vi "GetParameters.vi"(0 "Camera Reference in":refnum<k24>, 1 "error in (no error)":errorcluster) -> (2 "2D ExposureMode (Timed Auto HDR Flash)":enum16{"Timed", "Auto", "HDR", "Flash"}(ring), 3 "2D ExposureTime (0.1-999)":dbl=0.1 min=0.1 max=999.0 step=0.1, 4 "2D Gray Value":i32 min=1 max=999 step=1, 5 "2D Auto-Exposure ROI (x, y, width, height)":T2, 6 "2D Tone Mapping":bool, 7 "2D HDR Exposure Count":i32, 8 "2D HDR Exposure Sequence":T1, 9 "3D Exposure Multiplier":i32, 10 "3D Exposure Sequence":T3, 11 "3D Gain (0-16)":dbl, 12 "Depth Range (lower upper)":cluster{"lower":i32, "upper":i32}, 13 "ROI (x, y, width, height)":T2, 14 "Camera Reference out":refnum<k24>, 15 "error out":errorcluster, 16 "PointCloudSurfaceSmoothing (Off Weak Normal Strong)":u8(ring) items=["Off", "Weak", "Normal", "Strong"], 17 "PointCloudNoiseRemoval (Off Weak Normal Strong)":u8(ring) items=["Off", "Weak", "Normal", "Strong"], 18 "PointCloudOutlierRemoval (Off Weak Normal Strong)":u8(ring) items=["Off", "Weak", "Normal", "Strong"], 19 "Stripe Contrast Threshold (0-100)":i32 min=0 max=100 step=1)   [LabVIEW 2023]
uses:
  C:/Program Files/National Instruments/LabVIEW 2025/MechEyeApiNet.dll
  Program Files/National Instruments/LabVIEW 2025/MechEyeApiNet.dll
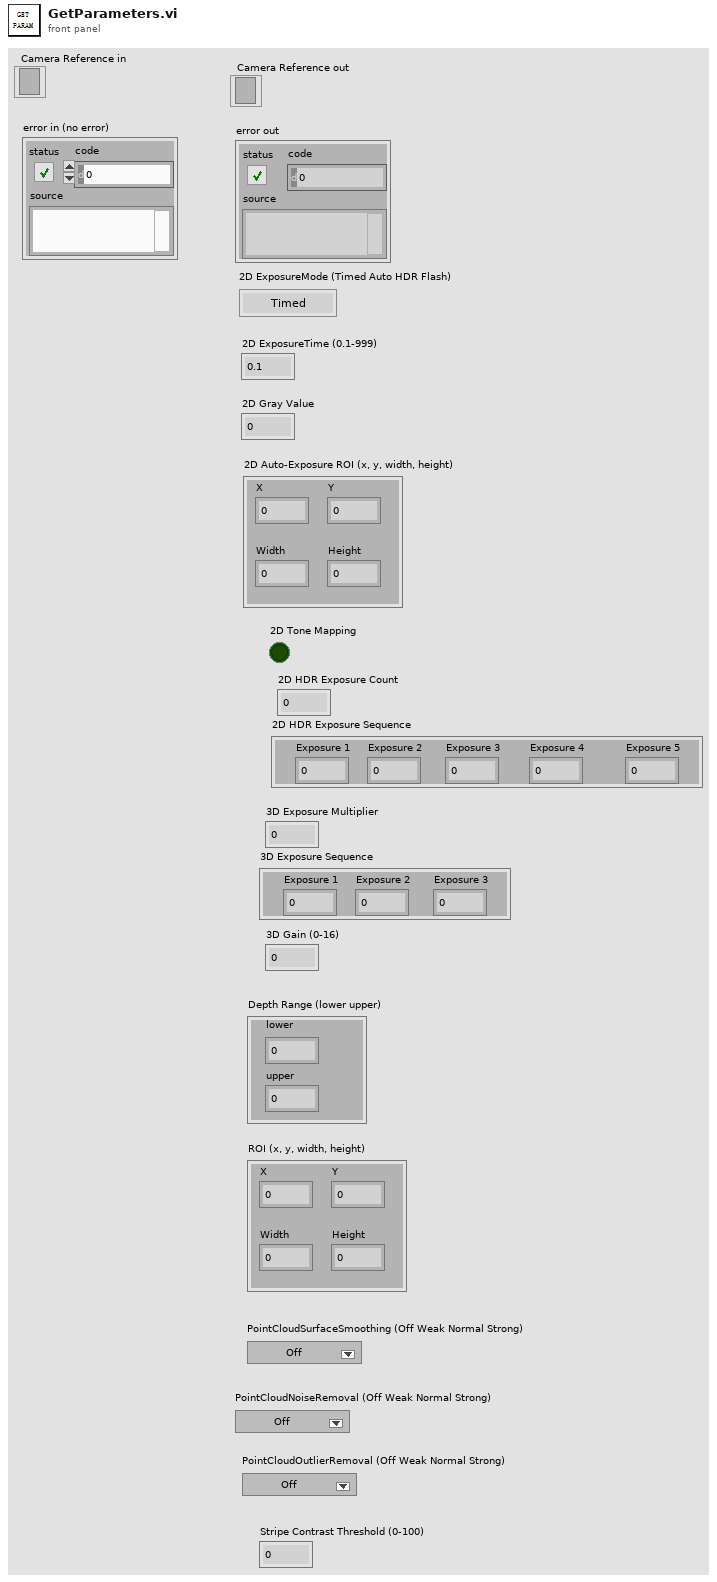
[diagram p1: front panel]
types:
  T1 = cluster{"Exposure 1":dbl, "Exposure 2":dbl, "Exposure 3":dbl, "Exposure 4":dbl, "Exposure 5":dbl}
  T2 = cluster{"X":i32, "Y":i32, "Width":i32, "Height":i32}
  T3 = cluster{"Exposure 1":dbl, "Exposure 2":dbl, "Exposure 3":dbl}
  T4 = cluster{"UpperLeftX":u32, "UpperLeftY":u32, "Width":u64, "Height":u64}
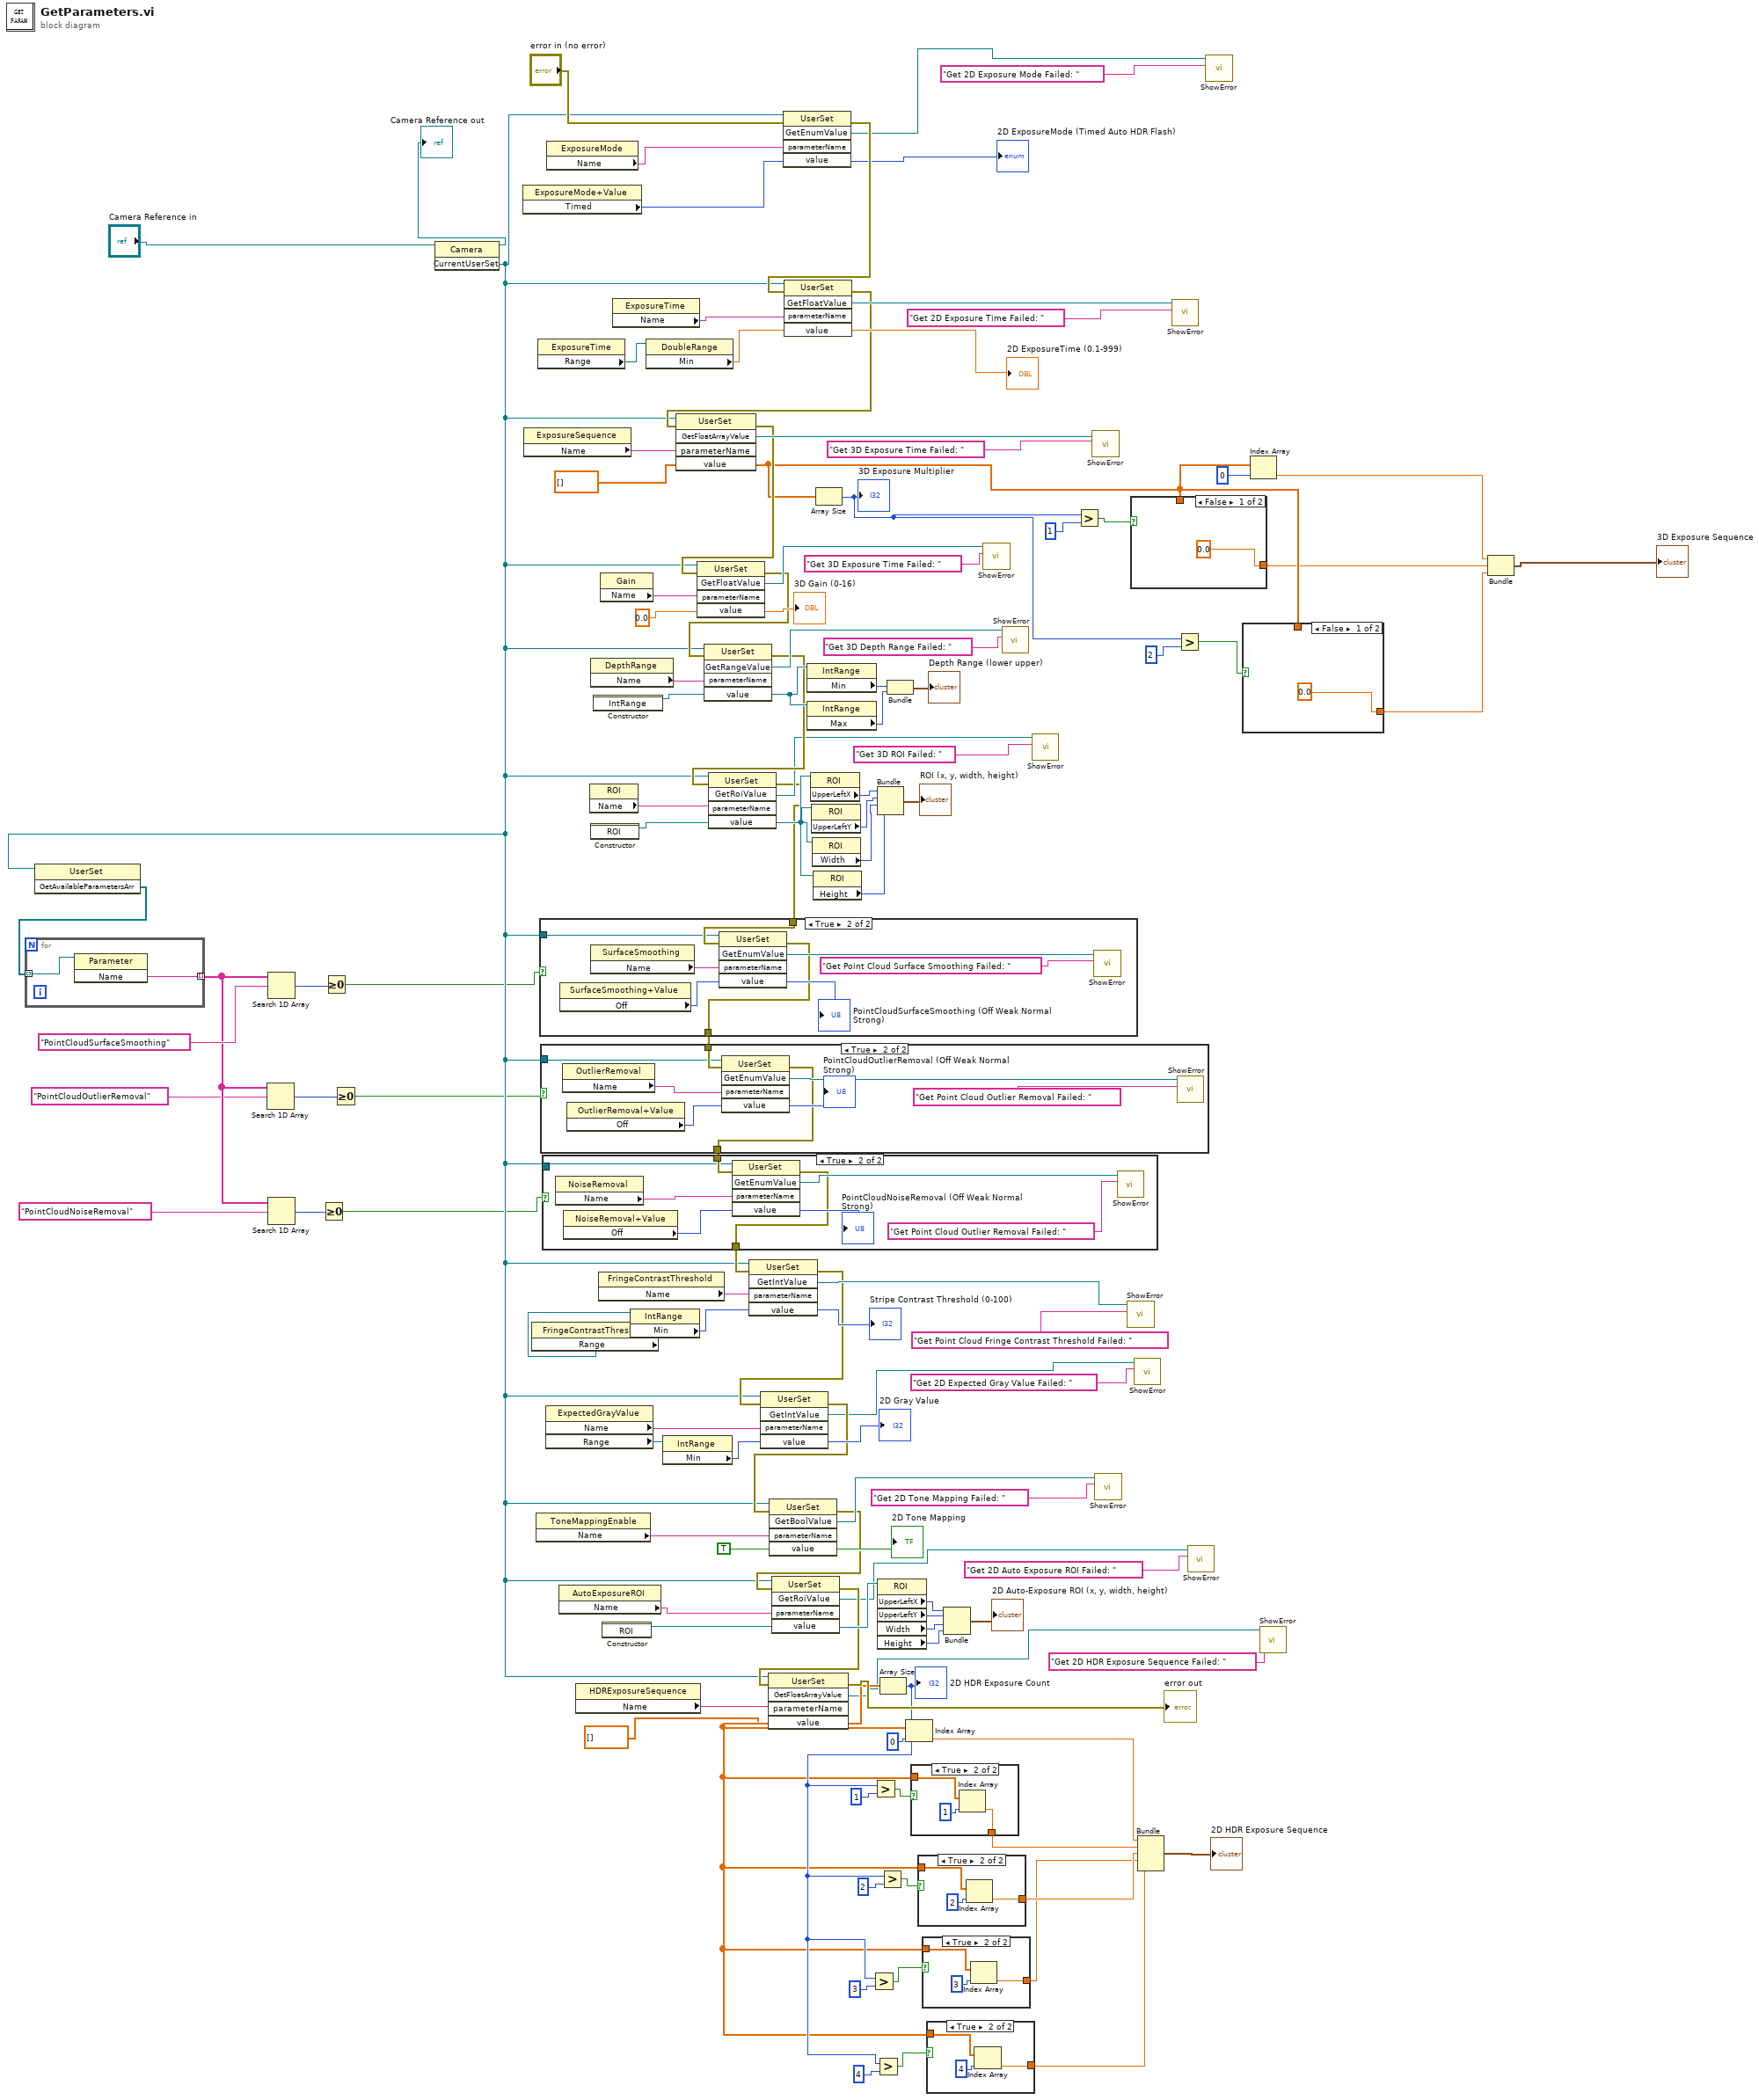
[diagram p0: block diagram]
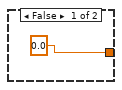
[diagram p5: hidden frame]
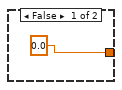
[diagram p6: hidden frame]
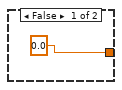
[diagram p7: hidden frame]
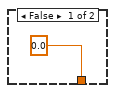
[diagram p8: hidden frame]
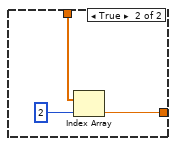
[diagram p9: hidden frame]
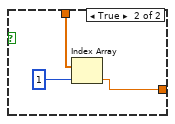
[diagram p10: hidden frame]
diagram:
  n1 = invoke class="Camera" method="CurrentUserSet"(reference="Camera Reference in") -> (reference out=→"Camera Reference out":refnum<k24>, "CurrentUserSet"=w12:refnum<k24>)  [unwired: 2 in, 1 out]
  n2 = invoke class="UserSet" method="GetAvailableParametersArr"(reference=w12) -> ("GetAvailableParametersArr"=w11:refnum<k24>[])  [unwired: 2 in, 2 out]
  n3 = for {
    tunnel: w11 -> [w128] mode=indexing
    tunnel: [w127] -> w7 mode=indexing
    n4 = invoke class="Parameter" method="Name"(reference=w128) -> ("Name"=w127:string)  [unwired: 2 in, 2 out]
  }
  n5 = Search 1D Array(1D array=w7, element="PointCloudOutlierRemoval") -> (index of element=w4:i32)  [unwired: 1 in]
  n6 = Search 1D Array(1D array=w7, element="PointCloudSurfaceSmoothing") -> (index of element=w9:i32)  [unwired: 1 in]
  n7 = Search 1D Array(1D array=w7, element="PointCloudNoiseRemoval") -> (index of element=w3:i32)  [unwired: 1 in]
  n8 = Greater Or Equal To 0?(x=w3) -> (x >= 0?=w1:bool)
  n9 = Greater Or Equal To 0?(x=w9) -> (x >= 0?=w8:bool)
  n10 = Greater Or Equal To 0?(x=w4) -> (x >= 0?=w2:bool)
  n11 = property class="ExposureMode+Value"() -> ("Timed"=w116:i32)  [unwired: 2 in, 2 out]
  n12 = property class="ExposureSequence"() -> ("Name"=w113:string)  [unwired: 2 in, 2 out]
  n13 = property class="FringeContrastThreshold"() -> ("Range"=w74:refnum<k24>)  [unwired: 2 in, 2 out]
  n14 = property class="ToneMappingEnable"() -> ("Name"=w53:string)  [unwired: 2 in, 2 out]
  n15 = property class="ExposureTime"() -> ("Range"=w115:refnum<k24>)  [unwired: 2 in, 2 out]
  n16 = property class="ExpectedGrayValue"() -> ("Name"=w57:string, "Range"=w56:refnum<k24>)  [unwired: 2 in, 2 out]
  n17 = property class="ExposureMode"() -> ("Name"=w120:string)  [unwired: 2 in, 2 out]
  n18 = property class="AutoExposureROI"() -> ("Name"=w45:string)  [unwired: 2 in, 2 out]
  n19 = property class="HDRExposureSequence"() -> ("Name"=w36:string)  [unwired: 2 in, 2 out]
  n20 = property class="ROI"() -> ("Name"=w93:string)  [unwired: 2 in, 2 out]
  n21 = property class="DepthRange"() -> ("Name"=w104:string)  [unwired: 2 in, 2 out]
  n22 = constructor class="ROI"() -> (reference out=w92:refnum<k24>)  [unwired: 3 in, 2 out]
  n23 = constructor class="IntRange"() -> (reference out=w103:refnum<k24>)  [unwired: 3 in, 2 out]
  n24 = property class="FringeContrastThreshold"() -> ("Name"=w75:string)  [unwired: 2 in, 2 out]
  n25 = property class="Gain"() -> ("Name"=w107:string)  [unwired: 2 in, 2 out]
  n26 = constructor class="ROI"() -> (reference out=w38:refnum<k24>)  [unwired: 3 in, 2 out]
  n27 = property class="ExposureTime"() -> ("Name"=w118:string)  [unwired: 2 in, 2 out]
  n28 = property class="IntRange"(reference=w74) -> ("Min"=w73:i32)  [unwired: 1 in, 2 out]
  n29 = property class="DoubleRange"(reference=w115) -> ("Min"=w114:dbl)  [unwired: 1 in, 2 out]
  n30 = property class="IntRange"(reference=w56) -> ("Min"=w55:i32)  [unwired: 1 in, 2 out]
  n31 = invoke class="UserSet" method="GetEnumValue"(reference=w12, error in="error in (no error)", "parameterName"=w120, "value"=w116) -> (error out=w125:errorcluster, "GetEnumValue"=w122:refnum<k24>, "value"=→"2D ExposureMode (Timed Auto HDR Flash)":i32)  [unwired: 1 in, 2 out]
  n32 = invoke class="UserSet" method="GetFloatValue"(reference=w12, error in=w125, "parameterName"=w118, "value"=w114) -> (error out=w96:errorcluster, "GetFloatValue"=w121:refnum<k24>, "value"=→"2D ExposureTime (0.1-999)":dbl)  [unwired: 1 in, 2 out]
  n33 = invoke class="UserSet" method="GetFloatArrayValue"(reference=w12, error in=w96, "parameterName"=w113, "value"=dbl[] [] ("Array")) -> (error out=w95:errorcluster, "GetFloatArrayValue"=w110:refnum<k24>, "value"=w66:dbl[])  [unwired: 1 in, 2 out]
  n34 = invoke class="UserSet" method="GetFloatValue"(reference=w12, error in=w95, "parameterName"=w107, "value"=0.0) -> (error out=w94:errorcluster, "GetFloatValue"=w105:refnum<k24>, "value"=→"3D Gain (0-16)":dbl)  [unwired: 1 in, 2 out]
  n35 = invoke class="UserSet" method="GetRangeValue"(reference=w12, error in=w94, "parameterName"=w104, "value"=w103) -> (error out=w91:errorcluster, "GetRangeValue"=w97:refnum<k24>, "value"=w102:refnum<k24>)  [unwired: 1 in, 2 out]
  n36 = invoke class="UserSet" method="GetRoiValue"(reference=w12, error in=w91, "parameterName"=w93, "value"=w92) -> (error out=w82:errorcluster, "GetRoiValue"=w83:refnum<k24>, "value"=w90:refnum<k24>)  [unwired: 1 in, 2 out]
  n37 = case shown="True" w8 {
    tunnel: w82 -> [w129 w132]
    tunnel: [w129 w131] -> w81
    tunnel: w12 -> [_ w130]
    frame False {
    }
    frame True {
      n38 = property class="SurfaceSmoothing+Value"() -> ("Off"=w135:i32)  [unwired: 2 in, 2 out]
      n39 = property class="SurfaceSmoothing"() -> ("Name"=w136:string)  [unwired: 2 in, 2 out]
      n40 = invoke class="UserSet" method="GetEnumValue"(reference=w130, error in=w132, "parameterName"=w136, "value"=w135) -> (error out=w131:errorcluster, "GetEnumValue"=w133:refnum<k24>, "value"=→"PointCloudSurfaceSmoothing (Off Weak Normal Strong)":i32)  [unwired: 1 in, 2 out]
      n41 = call "ShowError.vi"("String"="Get Point Cloud Surface Smoothing Failed: ", "MMind.Eye.ErrorStatus"=w133) -> ()  [unwired: 10 in]
    }
  }
  n42 = case shown="True" w2 {
    tunnel: w81 -> [w138 w141]
    tunnel: [w138 w140] -> w80
    tunnel: w12 -> [_ w139]
    frame False {
    }
    frame True {
      n43 = property class="OutlierRemoval"() -> ("Name"=w146:string)  [unwired: 2 in, 2 out]
      n44 = property class="OutlierRemoval+Value"() -> ("Off"=w145:i32)  [unwired: 2 in, 2 out]
      n45 = invoke class="UserSet" method="GetEnumValue"(reference=w139, error in=w141, "parameterName"=w146, "value"=w145) -> (error out=w140:errorcluster, "GetEnumValue"=w142:refnum<k24>, "value"=→"PointCloudOutlierRemoval (Off Weak Normal Strong)":i32)  [unwired: 1 in, 2 out]
      n46 = call "ShowError.vi"("String"="Get Point Cloud Outlier Removal Failed: ", "MMind.Eye.ErrorStatus"=w142) -> ()  [unwired: 10 in]
    }
  }
  n47 = case shown="True" w1 {
    tunnel: w80 -> [w147 w150]
    tunnel: [w147 w149] -> w78
    tunnel: w12 -> [_ w148]
    frame False {
    }
    frame True {
      n48 = property class="NoiseRemoval"() -> ("Name"=w155:string)  [unwired: 2 in, 2 out]
      n49 = property class="NoiseRemoval+Value"() -> ("Off"=w154:i32)  [unwired: 2 in, 2 out]
      n50 = invoke class="UserSet" method="GetEnumValue"(reference=w148, error in=w150, "parameterName"=w155, "value"=w154) -> (error out=w149:errorcluster, "GetEnumValue"=w151:refnum<k24>, "value"=→"PointCloudNoiseRemoval (Off Weak Normal Strong)":i32)  [unwired: 1 in, 2 out]
      n51 = call "ShowError.vi"("String"="Get Point Cloud Outlier Removal Failed: ", "MMind.Eye.ErrorStatus"=w151) -> ()  [unwired: 10 in]
    }
  }
  n52 = invoke class="UserSet" method="GetIntValue"(reference=w12, error in=w78, "parameterName"=w75, "value"=w73) -> (error out=w59:errorcluster, "GetIntValue"=w76:refnum<k24>, "value"=→"Stripe Contrast Threshold (0-100)":i32)  [unwired: 1 in, 2 out]
  n53 = invoke class="UserSet" method="GetIntValue"(reference=w12, error in=w59, "parameterName"=w57, "value"=w55) -> (error out=w51:errorcluster, "GetIntValue"=w49:refnum<k24>, "value"=→"2D Gray Value":i32)  [unwired: 1 in, 2 out]
  n54 = invoke class="UserSet" method="GetBoolValue"(reference=w12, error in=w51, "parameterName"=w53, "value"=TRUE) -> (error out=w46:errorcluster, "GetBoolValue"=w47:refnum<k24>, "value"=→"2D Tone Mapping":bool)  [unwired: 1 in, 2 out]
  n55 = invoke class="UserSet" method="GetRoiValue"(reference=w12, error in=w46, "parameterName"=w45, "value"=w38) -> (error out=w37:errorcluster, "GetRoiValue"=w15:refnum<k24>, "value"=w44:refnum<k24>)  [unwired: 1 in, 2 out]
  n56 = invoke class="UserSet" method="GetFloatArrayValue"(reference=w12, error in=w37, "parameterName"=w36, "value"=dbl[] []) -> (error out=→"error out":errorcluster, "GetFloatArrayValue"=w13:refnum<k24>, "value"=w19:dbl[])  [unwired: 1 in, 2 out]
  n57 = property class="IntRange"(reference=w102) -> ("Min"=w101:i32)  [unwired: 1 in, 2 out]
  n58 = property class="IntRange"(reference=w102) -> ("Max"=w100:i32)  [unwired: 1 in, 2 out]
  n59 = property class="ROI"(reference=w90) -> ("UpperLeftX"=w88:u32)  [unwired: 1 in, 2 out]
  n60 = property class="ROI"(reference=w90) -> ("UpperLeftY"=w87:u32)  [unwired: 1 in, 2 out]
  n61 = property class="ROI"(reference=w90) -> ("Width"=w86:u64)  [unwired: 1 in, 2 out]
  n62 = property class="ROI"(reference=w90) -> ("Height"=w85:u64)  [unwired: 1 in, 2 out]
  n63 = Array Size(array=w66) -> (size(s)=w68:i32)
  "3D Exposure Multiplier" <- w68
  n64 = Bundle("UpperLeftX"=w88, "UpperLeftY"=w87, "Width"=w86, "Height"=w85) -> (→"ROI (x, y, width, height)":T4)  [unwired: 1 in]
  n65 = property class="ROI"(reference=w44) -> ("UpperLeftX"=w42:u32, "UpperLeftY"=w41:u32, "Width"=w40:u64, "Height"=w39:u64)  [unwired: 1 in, 2 out]
  n66 = Array Size(array=w19) -> (size(s)=w20:i32)
  "2D HDR Exposure Count" <- w20
  n67 = Greater?(x=w20, y=3) -> (0:w24:bool)
  n68 = Greater?(x=w20, y=1) -> (0:w32:bool)
  n69 = Greater?(x=w20, y=4) -> (0:w21:bool)
  n70 = Greater?(x=w20, y=2) -> (0:w30:bool)
  n71 = Bundle("Min"=w101, "Max"=w100) -> (→"Depth Range (lower upper)":cluster{"Min":i32, "Max":i32})  [unwired: 1 in]
  n72 = Index Array(array=w19, index=0) -> (element=w28:dbl)
  n73 = case shown="True" w32 {
    tunnel: w19 -> [_ w158]
    tunnel: [0.0 w157] -> w27
    frame False {
    }
    frame True {
      n74 = Index Array(array=w158, index=1) -> (element=w157:dbl)
    }
  }
  n75 = case shown="True" w30 {
    tunnel: w19 -> [_ w162]
    tunnel: [0.0 w161] -> w26
    frame False {
    }
    frame True {
      n76 = Index Array(array=w162, index=2) -> (element=w161:dbl)
    }
  }
  n77 = case shown="True" w24 {
    tunnel: w19 -> [_ w166]
    tunnel: [0.0 w165] -> w23
    frame False {
    }
    frame True {
      n78 = Index Array(array=w166, index=3) -> (element=w165:dbl)
    }
  }
  n79 = case shown="True" w21 {
    tunnel: w19 -> [_ w170]
    tunnel: [0.0 w169] -> w18
    frame False {
    }
    frame True {
      n80 = Index Array(array=w170, index=4) -> (element=w169:dbl)
    }
  }
  n81 = Bundle("UpperLeftX"=w42, "UpperLeftY"=w41, "Width"=w40, "Height"=w39) -> (→"2D Auto-Exposure ROI (x, y, width, height)":T4)  [unwired: 1 in]
  n82 = call "ShowError.vi"("String"="Get 3D Exposure Time Failed: ", "MMind.Eye.ErrorStatus"=w105) -> ()  [unwired: 10 in]
  n83 = call "ShowError.vi"("String"="Get 3D Depth Range Failed: ", "MMind.Eye.ErrorStatus"=w97) -> ()  [unwired: 10 in]
  n84 = call "ShowError.vi"("String"="Get 3D ROI Failed: ", "MMind.Eye.ErrorStatus"=w83) -> ()  [unwired: 10 in]
  n85 = Greater?(x=w68, y=1) -> (0:w70:bool)
  n86 = call "ShowError.vi"("String"="Get 3D Exposure Time Failed: ", "MMind.Eye.ErrorStatus"=w110) -> ()  [unwired: 10 in]
  n87 = call "ShowError.vi"("String"="Get 2D Tone Mapping Failed: ", "MMind.Eye.ErrorStatus"=w47) -> ()  [unwired: 10 in]
  n88 = call "ShowError.vi"("String"="Get Point Cloud Fringe Contrast Threshold Failed: ", "MMind.Eye.ErrorStatus"=w76) -> ()  [unwired: 10 in]
  n89 = case shown="False" w70 {
    tunnel: w66 -> [_ w174]
    tunnel: [0.0 w173] -> w64
    frame False {
    }
    frame True {
      n90 = Index Array(array=w174, index=1) -> (element=w173:dbl)
    }
  }
  n91 = call "ShowError.vi"("String"="Get 2D Expected Gray Value Failed: ", "MMind.Eye.ErrorStatus"=w49) -> ()  [unwired: 10 in]
  n92 = Bundle(w28, w27, w26, w23, w18) -> (→"2D HDR Exposure Sequence":cluster{dbl, dbl, dbl, dbl, dbl})  [unwired: 1 in]
  n93 = call "ShowError.vi"("String"="Get 2D Exposure Time Failed: ", "MMind.Eye.ErrorStatus"=w121) -> ()  [unwired: 10 in]
  n94 = Greater?(x=w68, y=2) -> (0:w67:bool)
  n95 = call "ShowError.vi"("String"="Get 2D Auto Exposure ROI Failed: ", "MMind.Eye.ErrorStatus"=w15) -> ()  [unwired: 10 in]
  n96 = call "ShowError.vi"("String"="Get 2D Exposure Mode Failed: ", "MMind.Eye.ErrorStatus"=w122) -> ()  [unwired: 10 in]
  n97 = case shown="False" w67 {
    tunnel: w66 -> [_ w178]
    tunnel: [0.0 w177] -> w63
    frame False {
    }
    frame True {
      n98 = Index Array(array=w178, index=2) -> (element=w177:dbl)
    }
  }
  n99 = Index Array(array=w66, index=0) -> (element=w65:dbl)
  n100 = call "ShowError.vi"("String"="Get 2D HDR Exposure Sequence Failed: ", "MMind.Eye.ErrorStatus"=w13) -> ()  [unwired: 10 in]
  n101 = Bundle(w65, w64, w63) -> (→"3D Exposure Sequence":cluster{dbl, dbl, dbl})  [unwired: 1 in]
